vi "AsyncLaunch Configure Front Panel Layouts.vi"(8 "error in":errorcluster, 9 "VIs to exclude":string[](array[string]), 10 "close window when done? (F)":bool, 11 "application reference":refnum<vi>) -> (0 "error out":errorcluster)   [LabVIEW 2010, in "NI_SE_Config Front Panel Layout.lvlib"]
uses:
  NI_SE_Config Front Panel Layout.lvlib
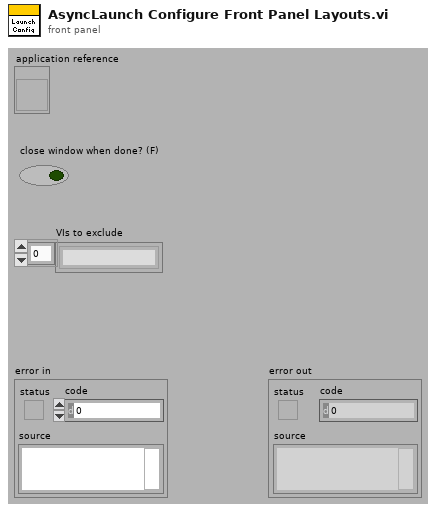
[diagram p1: front panel]
types:
  T1 = enum32{"Invalid", "Standard", "Closed", "Hidden", "Minimized", "Maximized"}
  T2 = enum32{"Bad", "Idle", "Run top level", "Running"}
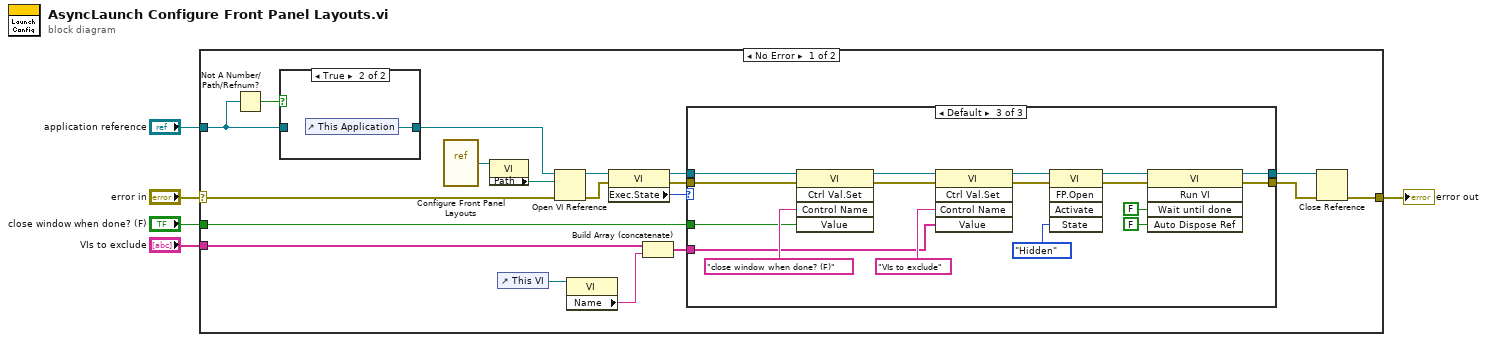
[diagram p0: block diagram]
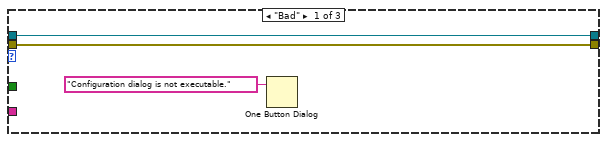
[diagram p2: hidden frame]
diagram:
  n1 = case shown="No Error" "error in" {
    selector: "error in" -> [w21 w49]
    tunnel: "application reference" -> [w20 _]
    tunnel: "close window when done? (F)" -> [w22 _]
    tunnel: "VIs to exclude" -> [w7 _]
    tunnel: [w17 w49] -> w1
    frame No Error {
      n2 = Not A Number/Path/Refnum?(number/path/refnum=w20) -> (NaN/Path/Refnum?=w18:bool)
      n3 = case shown="True" w18 {
        tunnel: [w47 w48] -> w19
        tunnel: w20 -> [w47 _]
        frame False {
        }
        frame True {
          n4 = control-ref of="This Application"() -> (w48:refnum<vi>)
        }
      }
      n5 = vi-ref "Configure Front Panel Layouts.vi"() -> (w24:refnum<vi>)
      n6 = property class="VI"(reference=w24) -> ("Path"=w23:path)  [unwired: 1 in, 2 out]
      n7 = control-ref of="This VI"() -> (w9:refnum<vi>)
      n8 = Open VI Reference(application reference (local)=w19, vi path=w23, error in (no error)=w21) -> (vi reference=w14:refnum<vi>, error out=w12:errorcluster)  [unwired: 3 in]
      n9 = property class="VI"(reference=w9) -> ("Name"=w8:string)  [unwired: 1 in, 2 out]
      n10 = property class="VI"(reference=w14, error in=w12) -> (reference out=w13:refnum<vi>, error out=w11:errorcluster, "Exec.State"=w10:T2)
      n11 = Build Array (concatenate)(w7, w8) -> (w6:string[])
      n12 = case shown="Default" w10 {
        tunnel: w22 -> [_ _ w45]
        tunnel: w6 -> [_ _ w41]
        tunnel: [w27 w28 w31] -> w16
        tunnel: [w26 w29 w30] -> w15
        tunnel: w13 -> [w27 w28 w38]
        tunnel: w11 -> [w26 w29 w37]
        frame "Bad" {
          n13 = One Button Dialog(message="Configuration dialog is not executable.") -> ()  [unwired: 1 in, 1 out]
        }
        frame "Run top level" {
        }
        frame Default {
          n14 = invoke class="VI" method="Ctrl Val.Set"(reference=w38, error in=w37, "Control Name"="close window when done? (F)", "Value"=w45) -> (reference out=w44:refnum<vi>, error out=w43:errorcluster)  [unwired: 1 in, 3 out]
          n15 = invoke class="VI" method="Ctrl Val.Set"(reference=w44, error in=w43, "Control Name"="VIs to exclude", "Value"=w41) -> (reference out=w35:refnum<vi>, error out=w33:errorcluster)  [unwired: 1 in, 3 out]
          n16 = invoke class="VI" method="FP.Open"(reference=w35, error in=w33, "State"=T1."Hidden") -> (reference out=w34:refnum<vi>, error out=w32:errorcluster)  [unwired: 2 in, 3 out]
          n17 = invoke class="VI" method="Run VI"(reference=w34, error in=w32, "Wait until done"=FALSE ("Wait Until Done"), "Auto Dispose Ref"=FALSE ("Auto Dispose Reference")) -> (reference out=w31:refnum<vi>, error out=w30:errorcluster)  [unwired: 1 in, 3 out]
        }
      }
      n18 = Close Reference(reference=w16, error in (no error)=w15) -> (error out=w17:errorcluster)
    }
    frame Error {
    }
  }
  "error out" <- w1
